vi "in_spline y2 to coefficients.vi"(9 "Y1":dbl[](array[numeric])=[1.7786639919453734e-13, -108.10714285714286, 72.42857142857147, -13.60714285714286, -5.696246425934692e-14], 10 "X":dbl[](array[numeric]), 11 "Y":dbl[](array[numeric])) -> (3 "coefficients":dbl[][](array[numeric]))   [LabVIEW 2020, in "NI_Gmath.lvlib"]
uses:
  NI_Gmath.lvlib
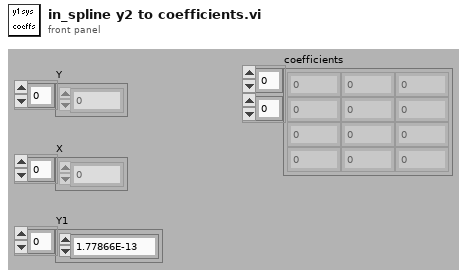
[diagram p1: front panel]
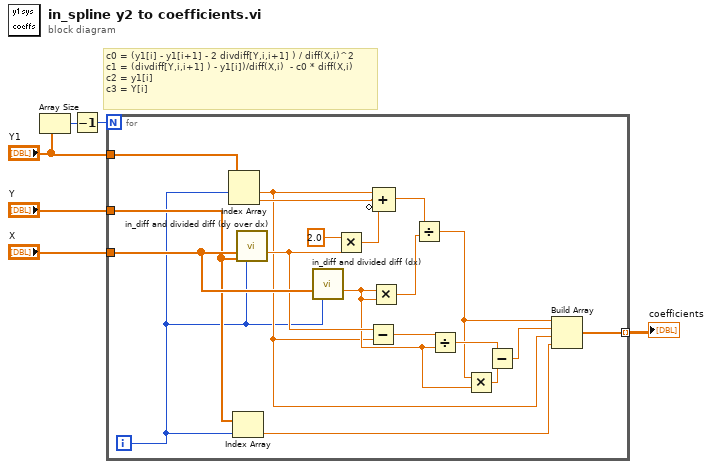
[diagram p0: block diagram]
diagram:
  # "c0 = (y1[i] - y1[i+1] - 2 divdiff[Y,i,i+1] ) / diff(X,i)^2\nc1 = (divdiff[Y,i,i+1] ) - y1[i])/diff(X,i)  - c0 * diff(X,i)\nc2 = y1[i]\nc3 = Y[i]"
  n1 = Array Size(array="Y1") -> (size(s)=w4:i32)
  n2 = Decrement(x=w4) -> (x-1=w3:i32)
  n3 = for {
    N: w3 -> [_]
    tunnel: "Y" -> [w10]
    tunnel: "X" -> [w21]
    tunnel: "Y1" -> [w25]
    tunnel: [w8] -> w1 mode=indexing
    i -> [w7]
    n4 = Index Array(array=w25, index #1=w7) -> (element #1=w11:dbl, element #2=w24:dbl)  [unwired: 1 in]
    n5 = Index Array(array=w10, index=w7) -> (element=w9:dbl)
    n6 = call "in_diff and divided diff (dy over dx).vi"("X"=w21, "Y"=w10, "i1"=w7) -> ("difference"=w18:dbl)  [unwired: 12 in]
    n7 = call "in_diff and divided diff (dx).vi"("X"=w21, "i1"=w7) -> ("difference"=w14:dbl)  [unwired: 13 in]
    n8 = Multiply(x=2.0, y=w18) -> (x*y=w22:dbl)
    n9 = Subtract(x=w18, y=w11) -> (x-y=w17:dbl)
    n10 = Multiply(x=w14, y=w14) -> (x*y=w19:dbl)
    n11 = Compound Arithmetic op=ADD(w11, w24, invert w22) -> (w20:dbl)
    n12 = Divide(x=w20, y=w19) -> (x/y=w15:dbl)
    n13 = Divide(x=w17, y=w14) -> (x/y=w16:dbl)
    n14 = Multiply(x=w15, y=w14) -> (x*y=w13:dbl)
    n15 = Subtract(x=w16, y=w13) -> (x-y=w12:dbl)
    n16 = Build Array(w15, w12, w11, w9) -> (w8:dbl[])
  }
  "coefficients" <- w1
